vi "create index groupings.vi"(8 "error in":errorcluster, 11 "data dictionary":refnum<class "data dictionary.lvclass">) -> (0 "error out":errorcluster, 2 "indices":T1[](array[typedef]))   [LabVIEW 2013, in "CVT runtime.lvclass"]
uses:
  CVT runtime.lvclass
  <vilib>/NI/Current Value Table/Type Defs/Typed Index Set.ctl
  <vilib>/NI/Current Value Table/Type Defs/Data Types.ctl
  <vilib>/NI/Tag Bus/dictionary/data dictionary.lvclass
  <vilib>/NI/Current Value Table/Type Defs/Single Tag.ctl
  <vilib>/NI/Current Value Table/Type Defs/File Format.ctl
  <vilib>/NI/Current Value Table/Type Defs/Tag Grouping set.ctl
  <vilib>/NI/Current Value Table/Errors/Generate Error.vi
  <vilib>/NI/Current Value Table/FGVs/Tag Memory.vi
  <vilib>/NI/Current Value Table/Current Value Table.lvlib
  configuration/CVT configuration.lvclass
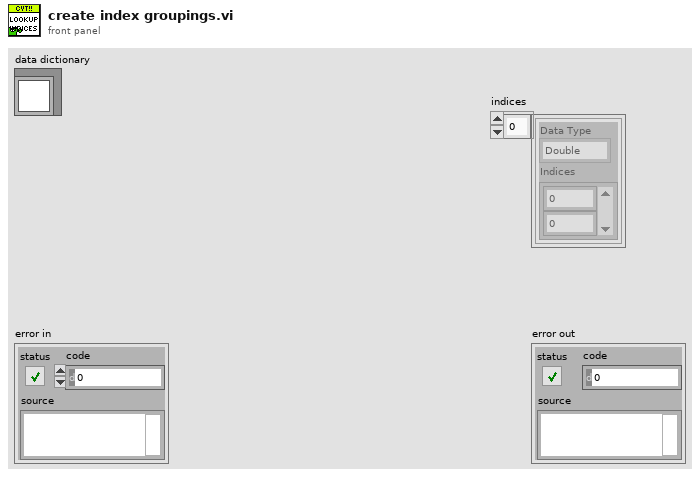
[diagram p1: front panel]
types:
  T1 = typedef "Current Value Table.lvlib/Typed Index Set.ctl" = cluster{"Data Type":T2, "Indices":i32[]}
  T2 = typedef "Current Value Table.lvlib/Data Types.ctl" = enum16{"Double", "Single", "I64", "I32", "I16", "I8", "U64", "U32", "U16", "U8", "String", "Boolean", "Array of U8", "Array of U16", "Array of U32", "Array of U64", "Array of I64", "Array of I32", "Array of I16", "Array of I8", "Array of Double", "Array of Single", "Array of Boolean", "Array of String"}
  T3 = typedef "tag bus.lvlib/tag descriptor.lvclass/Data Type.ctl" = enum16{"Double", "Single", "I64", "I32", "I16", "I8", "U64", "U32", "U16", "U8", "Boolean", "String", "Array of Double", "Array of Single", "Array of I64", "Array of I32", "Array of I16", "Array of I8", "Array of U64", "Array of U32", "Array of U16", "Array of U8", "Array of Boolean", "Array of String"}
  T4 = typedef "Current Value Table.lvlib/File Format.ctl" = cluster{"Tags":T5[], "Group Listings":T6[]}
  T5 = typedef "Current Value Table.lvlib/Single Tag.ctl" = cluster{"Data Type":T2, "Name":string, "Value":string, "Description":string}
  T6 = typedef "Current Value Table.lvlib/Tag Grouping set.ctl" = cluster{"Group":string, "Tag Names":string[]}
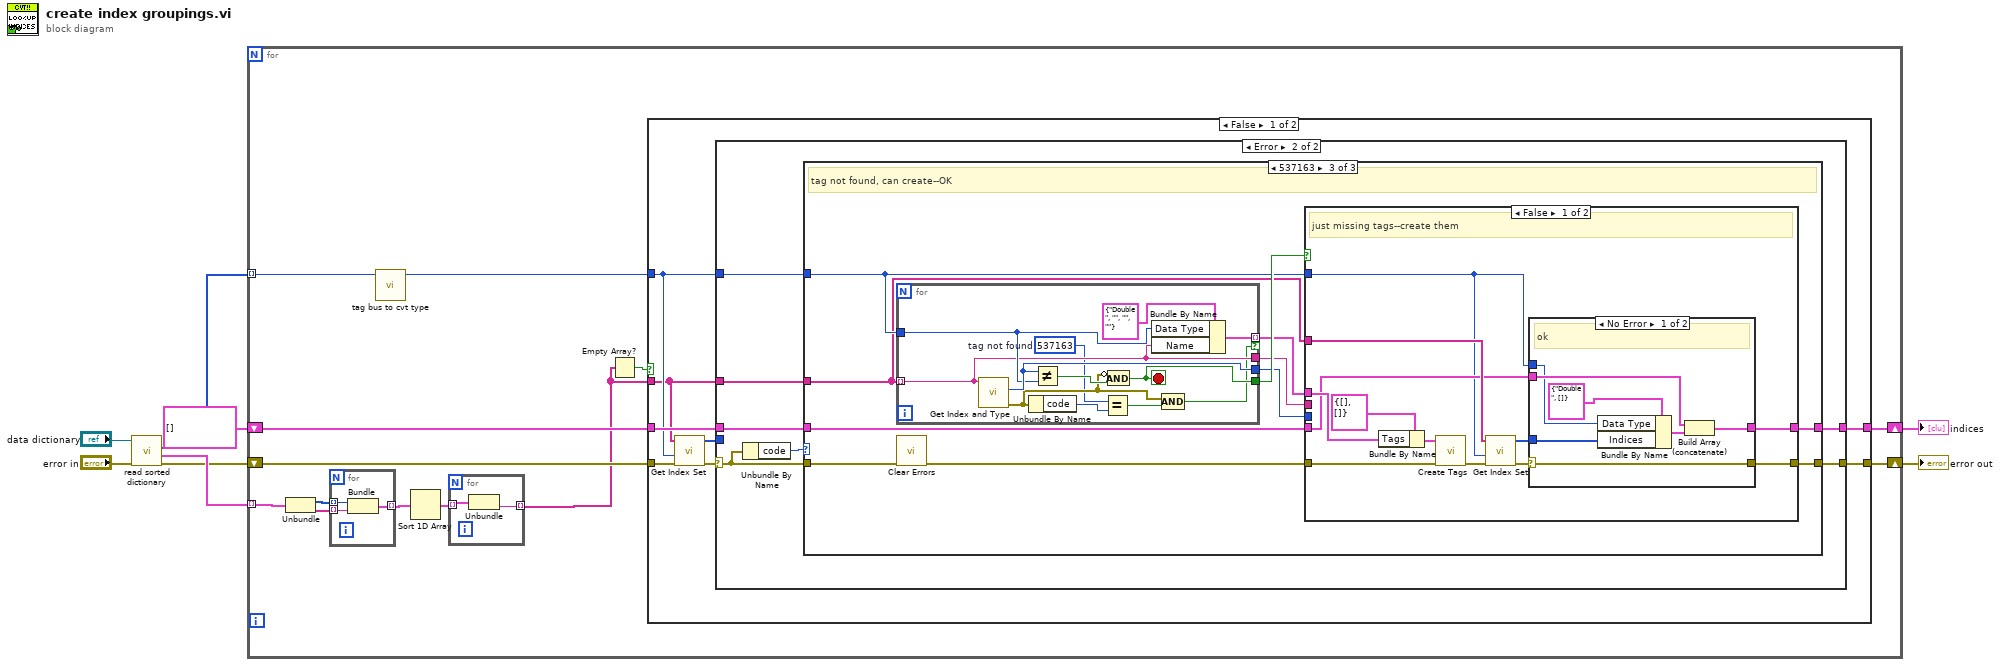
[diagram p0: block diagram]
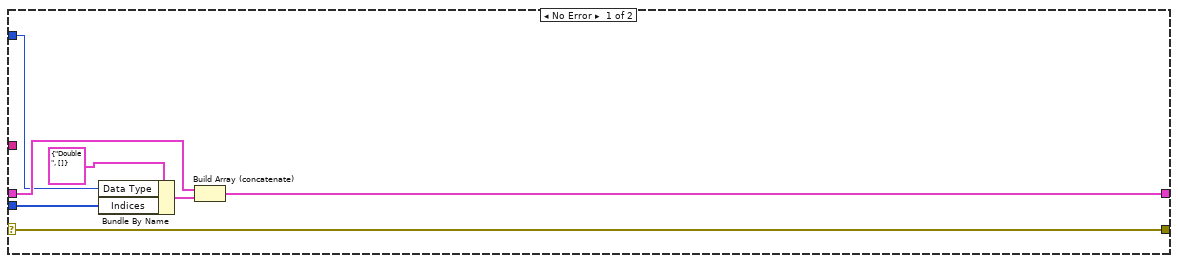
[diagram p2: hidden frame]
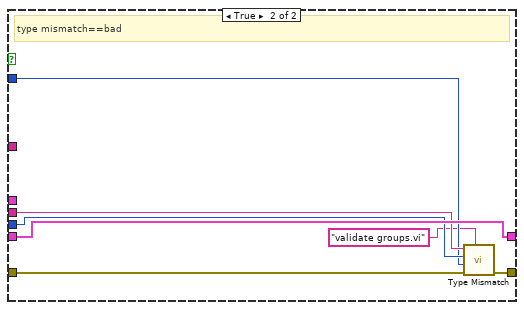
[diagram p6: hidden frame]
diagram:
  n1 = call <vilib>:"read sorted dictionary.vi"("error in"="error in", "data dictionary in"="data dictionary") -> ("error out"=w3:errorcluster, "tags by type"=w4:cluster{"indices":i32[], "names":string[]}[], "types"=w5:T3[])  [unwired: 6 in, 1 out]
  n2 = for {
    shift-right: [w21] -> w7
    shift-left: T1[] [] -> [w20]
    shift-right: [w18] -> w8
    shift-left: w3 -> [w19]
    tunnel: w5 -> [w15] mode=indexing
    tunnel: w4 -> [w14] mode=indexing
    n3 = Unbundle(w14) -> ("indices"=w13:i32[], "names"=w12:string[])
    n4 = for {
      tunnel: w13 -> [w26] mode=indexing
      tunnel: w12 -> [w25] mode=indexing
      tunnel: [w24] -> w11 mode=indexing
      n5 = Bundle(w26, "names"=w25) -> (w24:cluster{i32, "names":string})  [unwired: 1 in]
    }
    n6 = call "tag bus to cvt type.vi"("Data Type"=w15) -> ("cvt type"=w16:T2)  [unwired: 10 in]
    n7 = Sort 1D Array(array=w11) -> (sorted array=w10:cluster{i32, "names":string}[])
    n8 = for {
      tunnel: w10 -> [w23] mode=indexing
      tunnel: [w22] -> w9 mode=indexing
      n9 = Unbundle(w23) -> ("names"=w22:string)  [unwired: 1 out]
    }
    n10 = Empty Array?(array=w9) -> (empty?=w17:bool)
    n11 = case shown="False" w17 {
      tunnel: [w34 w105] -> w21
      tunnel: w20 -> [w33 w105]
      tunnel: w19 -> [w32 w104]
      tunnel: [w31 w104] -> w18
      tunnel: w16 -> [w28 _]
      tunnel: w9 -> [w27 _]
      frame False {
        n12 = call <vilib>:"Get Index Set.vi"("error in (no error)"=w32, "Expected Type"=w28, "Tag Names"=w27) -> ("error out"=w30:errorcluster, "Tag References"=w29:i32[])  [unwired: 7 in]
        n13 = case shown="Error" w30 {
          selector: w30 -> [w41 w44]
          tunnel: [w41 w45] -> w31
          tunnel: w33 -> [w39 w47]
          tunnel: [w38 w46] -> w34
          tunnel: w28 -> [w36 w42]
          tunnel: w29 -> [w35 _]
          tunnel: w27 -> [_ w43]
          frame No Error {
            n14 = Bundle By Name(cluster=T1 {"Data Type"=enum."Double", "Indices"=[]} ("Index Type Set"), "Data Type"=w36, "Indices"=w35) -> (w37:T1)
            n15 = Build Array (concatenate)(w39, w37) -> (w38:T1[])
          }
          frame Error {
            n16 = Unbundle By Name(w44) -> ("code"=w48:i32)
            n17 = case shown="537163" w48 {
              tunnel: w47 -> [w49 w52 w59]
              tunnel: [w49 w52 w60] -> w46
              tunnel: [w50 w51 w61] -> w45
              tunnel: w44 -> [w50 w51 w63]
              tunnel: w43 -> [_ _ w53]
              tunnel: w42 -> [_ _ w55]
              frame Default {
                # "unk"
              }
              frame 537165 {
                # "tag found but type mismatch"
              }
              frame 537163 {
                # "tag not found, can create--OK"
                n18 = for {
                  tunnel: w53 -> [w97] mode=indexing
                  tunnel: w55 -> [w98]
                  tunnel: [w102] -> w58
                  tunnel: [w97] -> w57
                  tunnel: [w101] -> w56
                  tunnel: [w99] -> w54 mode=indexing if=w92
                  stop <- w102 stop-if-true
                  w93 = 537163  # tag not found
                  n19 = call <vilib>:"Get Index and Type.vi"("Tag"=w97) -> ("error out"=w94:errorcluster, "Type"=w101:T2)  [unwired: 8 in, 1 out]
                  n20 = Unbundle By Name(w94) -> ("code"=w96:i32)
                  n21 = Not Equal?(x=w101, y=w98) -> (x != y?=w103:bool)
                  n22 = Equal?(x=w93, y=w96) -> (x = y?=w95:bool)
                  n23 = Compound Arithmetic op=AND(invert w94, w103) -> (w102:bool)
                  n24 = Bundle By Name(cluster=T5 {"Data Type"=enum."Double", "Name"="", "Value"="", "Description"=""} ("Tag"), "Data Type"=w98, "Name"=w97) -> (w99:T5)
                  n25 = Compound Arithmetic op=AND(w94, w95) -> (w92:bool)
                }
                n26 = call <vilib>:"Clear Errors.vi"("error in (no error)"=w63) -> ("error out"=w62:errorcluster)  [unwired: 6 in]
                n27 = case shown="False" w58 {
                  tunnel: w62 -> [w75 w91]
                  tunnel: [w71 w90] -> w61
                  tunnel: [w66 w89] -> w60
                  tunnel: w59 -> [w67 w89]
                  tunnel: w57 -> [_ w88]
                  tunnel: w56 -> [_ w87]
                  tunnel: w55 -> [w65 w86]
                  tunnel: w54 -> [w72 _]
                  tunnel: w53 -> [w69 _]
                  frame False {
                    # "just missing tags--create them"
                    n28 = Bundle By Name(cluster=T4 {"Tags"=[], "Group Listings"=[]} ("CVT Tags to Create"), "Tags"=w72) -> (w73:T4)
                    n29 = call <vilib>:"Create Tags.vi"("error in (no error)"=w75, "CVT Tags to Create"=w73) -> ("error out"=w70:errorcluster)  [unwired: 9 in]
                    n30 = call <vilib>:"Get Index Set.vi"("error in (no error)"=w70, "Expected Type"=w65, "Tag Names"=w69) -> ("error out"=w68:errorcluster, "Tag References"=w64:i32[])  [unwired: 7 in]
                    n31 = case shown="No Error" w68 {
                      selector: w68 -> [w82 w84]
                      tunnel: [w82 w84] -> w71
                      tunnel: w67 -> [w79 w83]
                      tunnel: [w78 w83] -> w66
                      tunnel: w65 -> [w77 _]
                      tunnel: w64 -> [w76 _]
                      frame No Error {
                        # "ok"
                        n32 = Bundle By Name(cluster=T1 {"Data Type"=enum."Double", "Indices"=[]} ("Index Type Set"), "Data Type"=w77, "Indices"=w76) -> (w80:T1)
                        n33 = Build Array (concatenate)(w79, w80) -> (w78:T1[])
                      }
                      frame Error {
                        # "unk"
                      }
                    }
                  }
                  frame True {
                    # "type mismatch==bad"
                    n34 = call <vilib>:"Type Mismatch.vi"("caller name"="validate groups.vi", "error in (no error)"=w91, "Data Type Requested"=w86, "True Type"=w87, "Tag"=w88) -> ("error out"=w90:errorcluster)  [unwired: 6 in]
                  }
                }
              }
            }
          }
        }
      }
      frame True {
      }
    }
  }
  "error out" <- w8
  "indices" <- w7
